vi "Flatten Time to String.vi"(8 "error in (no error)":errorcluster, 11 "Save Image in":refnum<class "Save Image.lvclass">) -> (0 "error out":errorcluster, 2 "flattened string":string, 3 "Save Image out":refnum<class "Save Image.lvclass">)   [LabVIEW 2018, in "Save Image.lvclass"]
uses:
  Save Image.lvclass
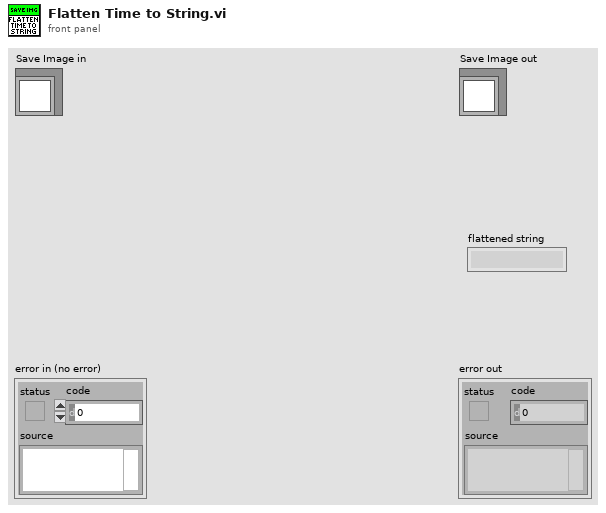
[diagram p1: front panel]
types:
  T1 = typedef "LVDateTimeRec.ctl" = cluster{"fractional second":dbl, "second":i32, "minute":i32, "hour":i32, "day of month":i32, "month":i32, "year":i32, "day of week":i32, "day of year":i32, "DST":i32}
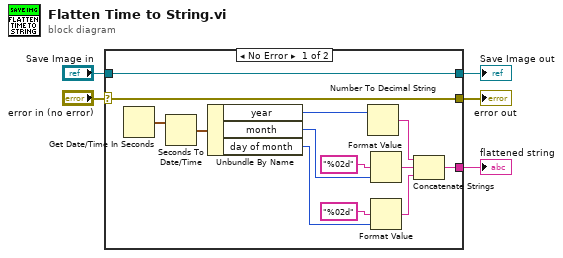
[diagram p0: block diagram]
diagram:
  n1 = case shown="No Error" "error in (no error)" {
    selector: "error in (no error)" -> [w17 w20]
    tunnel: [w17 w20] -> w4
    tunnel: [w18 w19] -> w2
    tunnel: "Save Image in" -> [w18 w19]
    tunnel: [w6 _] -> w1
    frame No Error {
      n2 = Get Date/Time In Seconds() -> (seconds since 1Jan1904=w11:timestamp)
      n3 = Seconds To Date/Time(time stamp (now)=w11) -> (date time rec=w10:T1)  [unwired: 1 in]
      n4 = Unbundle By Name(w10) -> ("year"=w16:i32, "month"=w13:i32, "day of month"=w12:i32)
      n5 = Number To Decimal String(number=w16) -> (decimal integer string=w9:string)  [unwired: 1 in]
      n6 = Format Value(format string="%02d", value (0)=w13) -> (output string=w8:string)  [unwired: 1 in]
      n7 = Format Value(format string="%02d", value (0)=w12) -> (output string=w7:string)  [unwired: 1 in]
      n8 = Concatenate Strings(w9, w8, w7) -> (w6:string)
    }
    frame Error {
    }
  }
  "error out" <- w4
  "Save Image out" <- w2
  "flattened string" <- w1
